vi "Запись в таблицу (SubVI).vi"(1 "data num":u32, 5 "error in":errorcluster, 6 "String Arr in":string[][](array[string]), 7 "Z axis data":dbl, 8 "Шаг измерений":u64, 9 "Y axis data":dbl, 11 "X axis data":dbl) -> (10 "String Arr out":string[][](array[string]), 14 "X axis data out":dbl, 15 "Y axis data out":dbl, 16 "Z axis data out":dbl, 19 "error out":errorcluster)   [LabVIEW 2013]
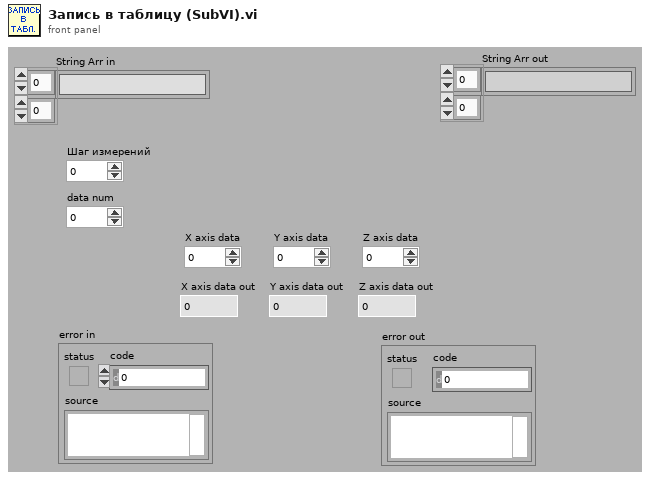
[diagram p1: front panel]
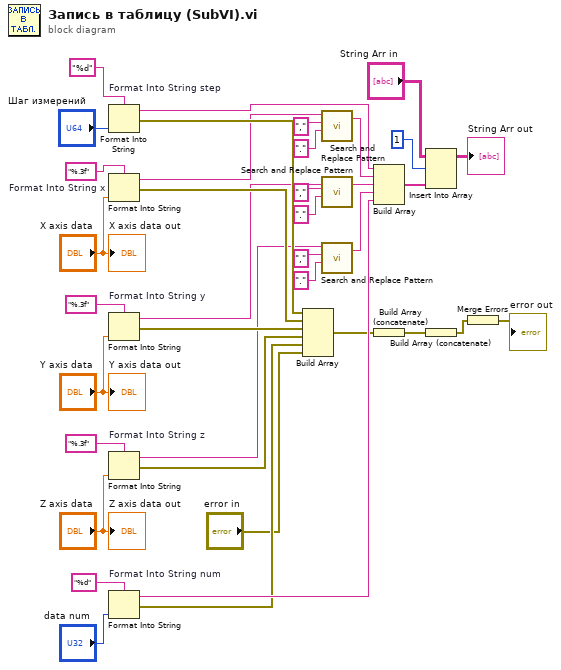
[diagram p0: block diagram]
diagram:
  n1 = Format Into String "Format Into String step"(format string="%d", "Шаг измерений") -> (resulting string=w24:string, error out=w21:errorcluster)  [unwired: 2 in]
  n2 = Format Into String "Format Into String x"(format string="%.3f", "X axis data") -> (resulting string=w10:string, error out=w20:errorcluster)  [unwired: 2 in]
  n3 = Format Into String "Format Into String y"(format string="%.3f", "Y axis data") -> (resulting string=w6:string, error out=w19:errorcluster)  [unwired: 2 in]
  n4 = Format Into String "Format Into String z"(format string="%.3f", "Z axis data") -> (resulting string=w1:string, error out=w18:errorcluster)  [unwired: 2 in]
  n5 = Format Into String "Format Into String num"(format string="%d", "data num") -> (resulting string=w23:string, error out=w17:errorcluster)  [unwired: 2 in]
  n6 = Build Array(w21, w20, w19, w18, w17, "error in") -> (w15:errorcluster[])
  n7 = call <vilib>:"Search and Replace Pattern.vi"("string"=w10, "regular expression (\"\")"="," ("regular expression (\"\")"), "replace string (\"\")"="." ("replace string (\"\")")) -> ("result string"=w9:string)  [unwired: 3 out]
  n8 = call <vilib>:"Search and Replace Pattern.vi"("string"=w6, "regular expression (\"\")"="," ("regular expression (\"\")"), "replace string (\"\")"="." ("replace string (\"\")")) -> ("result string"=w5:string)  [unwired: 3 out]
  n9 = call <vilib>:"Search and Replace Pattern.vi"("string"=w1, "regular expression (\"\")"="," ("regular expression (\"\")"), "replace string (\"\")"="." ("replace string (\"\")")) -> ("result string"=w2:string)  [unwired: 3 out]
  n10 = Build Array(w24, w9, w5, w2, w23) -> (w22:string[])
  n11 = Build Array (concatenate)(w15) -> (w14:errorcluster[])
  n12 = Insert Into Array(array="String Arr in", index (row)=1 ("disabled index (col)"), new element=w22) -> (→"String Arr out":string[][])  [unwired: 1 in]
  n13 = Build Array (concatenate)(w14) -> (w13:errorcluster[])
  n14 = Merge Errors(w13) -> (→"error out":errorcluster)
  "X axis data out" <- "X axis data"
  "Y axis data out" <- "Y axis data"
  "Z axis data out" <- "Z axis data"
